vi "参数配置表.vi"() -> ()   [LabVIEW 2016, in "数据传输系统.lvlib"]
uses:
  <vilib>/Utility/miscctls.llb/LVPointTypeDef.ctl
  <vilib>/Utility/config.llb/NI_LVConfig.lvlib
  <vilib>/ptbypt/NI_PtbyPt.lvlib
panel:
  in  "应用环境":enum16{"STD", "GB212"}(ring)
  in  "屏蔽维护数据":bool
  in  "数据发送延时时间/s":i32
  in  "判断数据反馈":enum16{"非严格判断", "严格判断", "不判断"}(ring)
  in  "仪器参数发送":bool
  in  "地表水/污染源":bool
  in  "等时间间隔分钟":i32
  in  "数据发送通道":enum16{"TCP", "VISA"}(ring)
  in  "数据发送协议":enum16{"2005-212协议", "2017-212协议"}(ring)=enum."2017-212协议"
  in  "数据触发上传方式":enum16{"出数即刻发送", "等时间间隔定时发送", "整点发送"}(ring)
  in  "数据组合发送":bool
  in  "日志、参数发送":bool
  in  "2011发送":bool
  in  "返回":bool
  out "配置表格":string[][](table)
  in  "参数数值":T1={"CODMn"=TRUE, "CODCr"=TRUE, "DO"=TRUE, "铜"=TRUE, "PH"=TRUE, "氨氮"=TRUE, "比电导率"=TRUE, "水温"=TRUE, "COD"=TRUE, "浊度"=TRUE, "总氮"=TRUE, "总磷"=TRUE, "叶绿素a"=TRUE, "藻密度"=TRUE, "水位"=TRUE, "流速"=TRUE, "瞬时流量"=TRUE, "累积流量"=TRUE, "亚硝氮"=TRUE, "硫化物"=TRUE, "ORP"=TRUE, "铅"=TRUE, "镉"=TRUE, "锌"=TRUE, "镍"=TRUE, "锰"=TRUE, "汞"=TRUE, "气温"=TRUE, "气压"=TRUE, "风速"=TRUE, "风向"=TRUE}
  # "因子编码，单位配置，上传功能码，小时、质控数据上传触发方式"
  # "参数配置"
  # "只对2017版出数即刻发送有效"
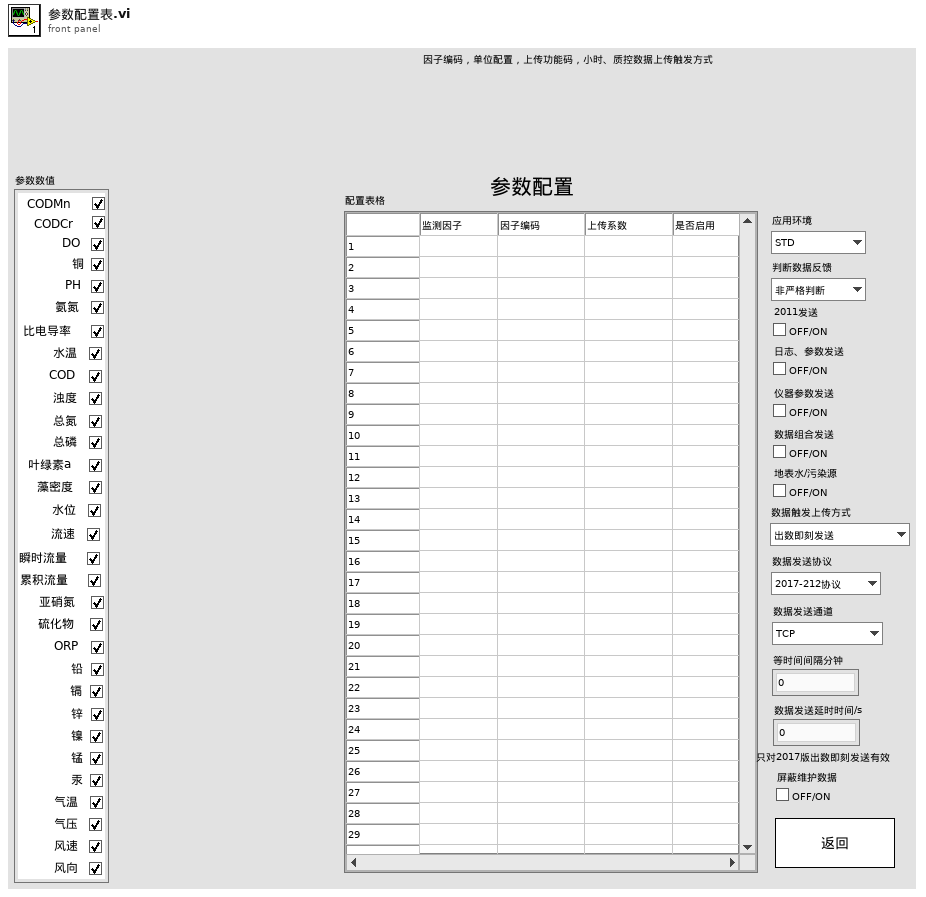
[diagram p1: front panel]
types:
  T1 = cluster{"CODMn":bool, "CODCr":bool, "DO":bool, "铜":bool, "PH":bool, "氨氮":bool, "比电导率":bool, "水温":bool, "COD":bool, "浊度":bool, "总氮":bool, "总磷":bool, "叶绿素a":bool, "藻密度":bool, "水位":bool, "流速":bool, "瞬时流量":bool, "累积流量":bool, "亚硝氮":bool, "硫化物":bool, "ORP":bool, "铅":bool, "镉":bool, "锌":bool, "镍":bool, "锰":bool, "汞":bool, "气温":bool, "气压":bool, "风速":bool, "风向":bool}
  T2 = typedef "LVPointTypeDef.ctl" = cluster{"Horizontal":i16, "Vertical":i16}
  T3 = typedef "NI_LVConfig.lvlib/Config Data RefNum.ctl" = refnum<k1>
  T4 = cluster{"[0]":string, "[1]":string, "[2]":string, "[3]":string, "[4]":string, "[5]":string, "[6]":string, "[7]":string, "[8]":string, "[9]":string, "[10]":string, "[11]":string, "[12]":string, "[13]":string, "[14]":string, "[15]":string, "[16]":string, "[17]":string, "[18]":string, "[19]":string, "[20]":string, "[21]":string, "[22]":string, "[23]":string, "[24]":string, "[25]":string, "[26]":string, "[27]":string, "[28]":string, "[29]":string, "[30]":string}
  T5 = enum8{"Enabled", "Disabled", "Disabled and Grayed Out"}
  T6 = typedef "LVRowAndColumnTypeDef.ctl" = cluster{"Row":i32, "Column":i32}
  T7 = cluster{"[0]":string, "[1]":string, "[2]":string, "[3]":string, "[4]":string, "[5]":string}
  T8 = cluster{"[0]":string, "[1]":string, "[2]":string, "[3]":string, "[4]":string, "[5]":string, "[6]":string, "[7]":string, "[8]":string, "[9]":string, "[10]":string, "[11]":string}
  T9 = cluster{"[0]":string, "[1]":string, "[2]":string, "[3]":string, "[4]":string, "[5]":string, "[6]":string, "[7]":string, "[8]":string, "[9]":string, "[10]":string, "[11]":string, "[12]":string}
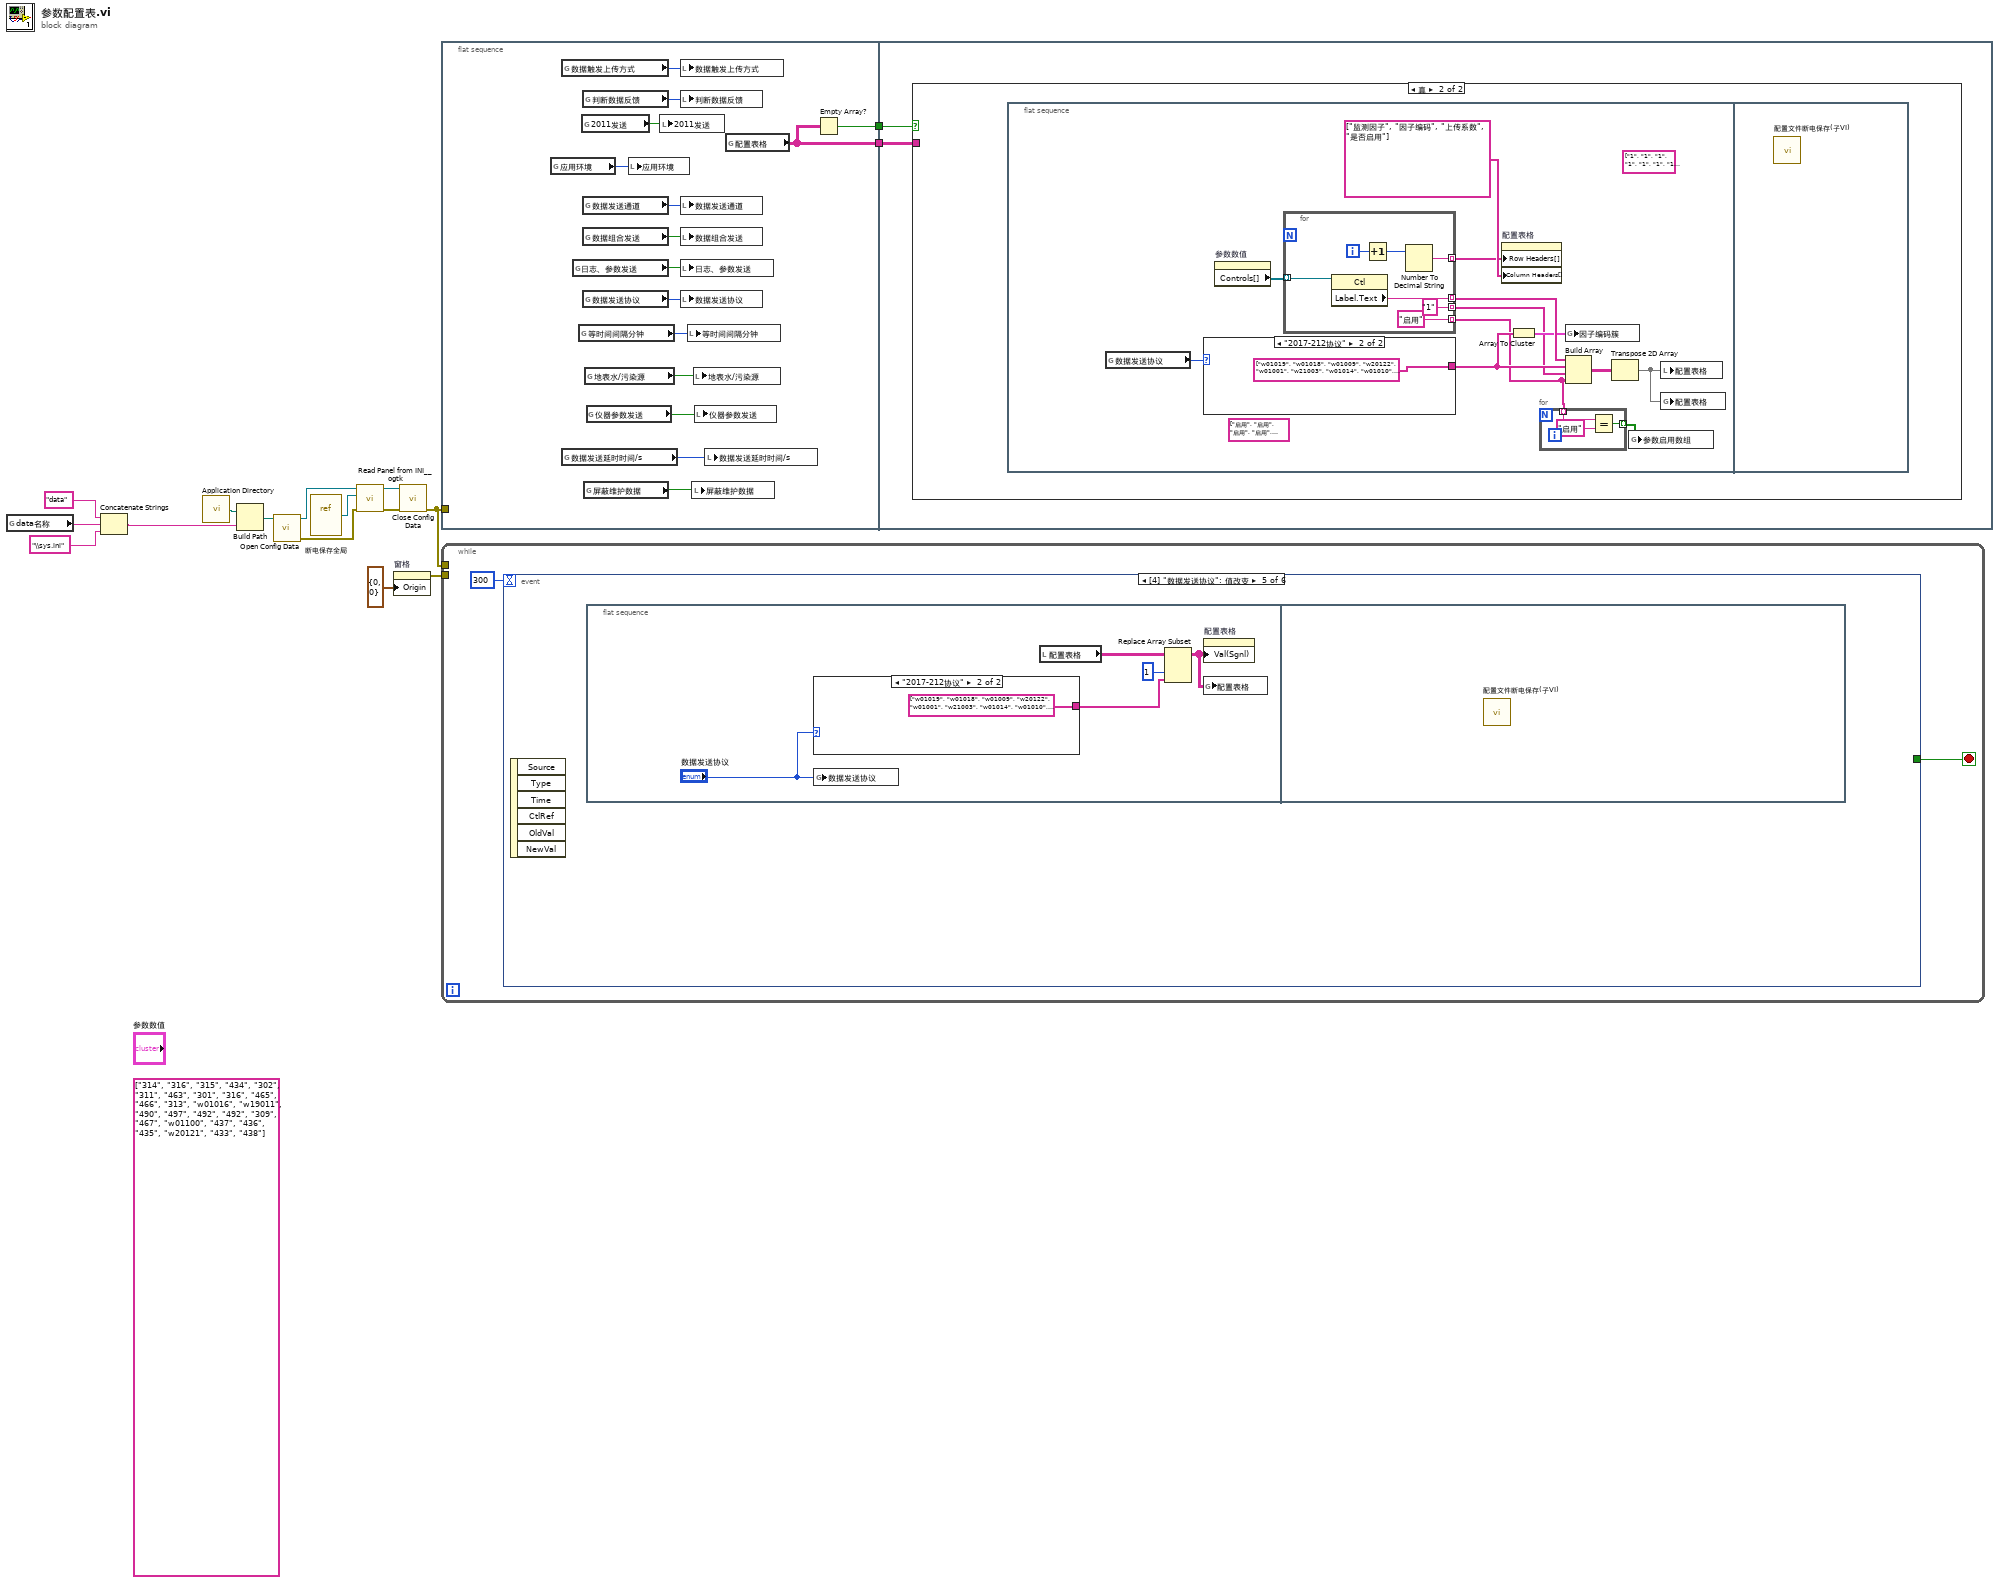
[diagram p0: block diagram]
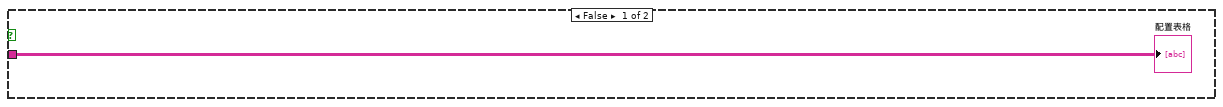
[diagram p2: hidden frame]
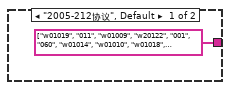
[diagram p3: hidden frame]
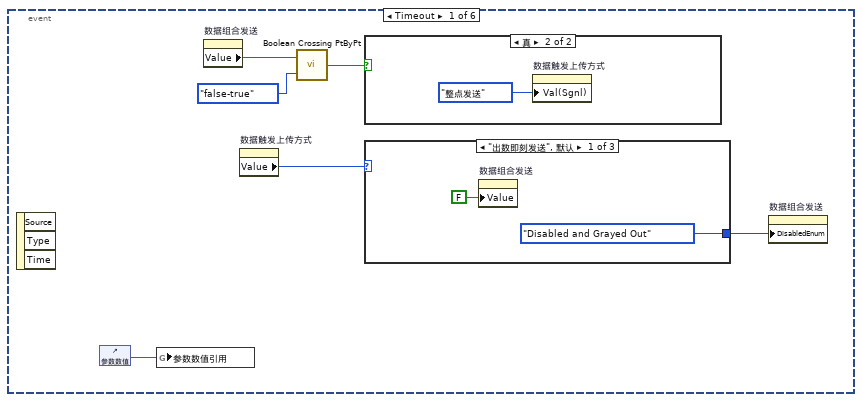
[diagram p4: hidden frame]
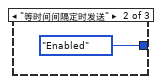
[diagram p6: hidden frame]
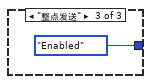
[diagram p7: hidden frame]
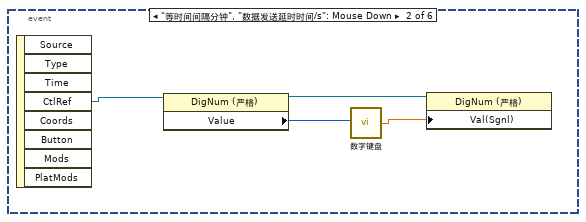
[diagram p8: hidden frame]
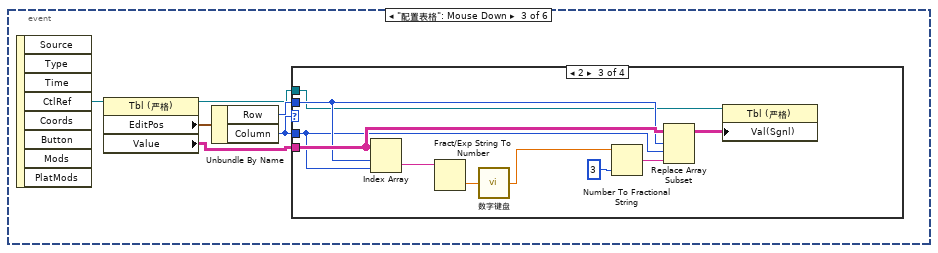
[diagram p9: hidden frame]
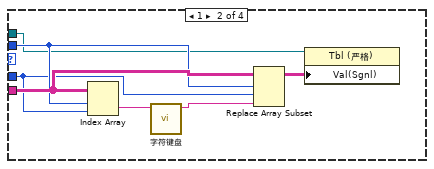
[diagram p11: hidden frame]
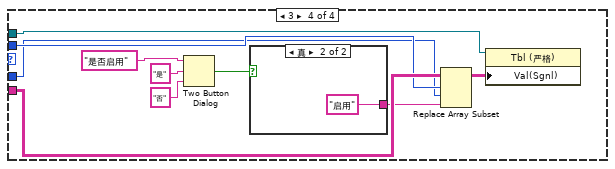
[diagram p12: hidden frame]
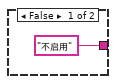
[diagram p13: hidden frame]
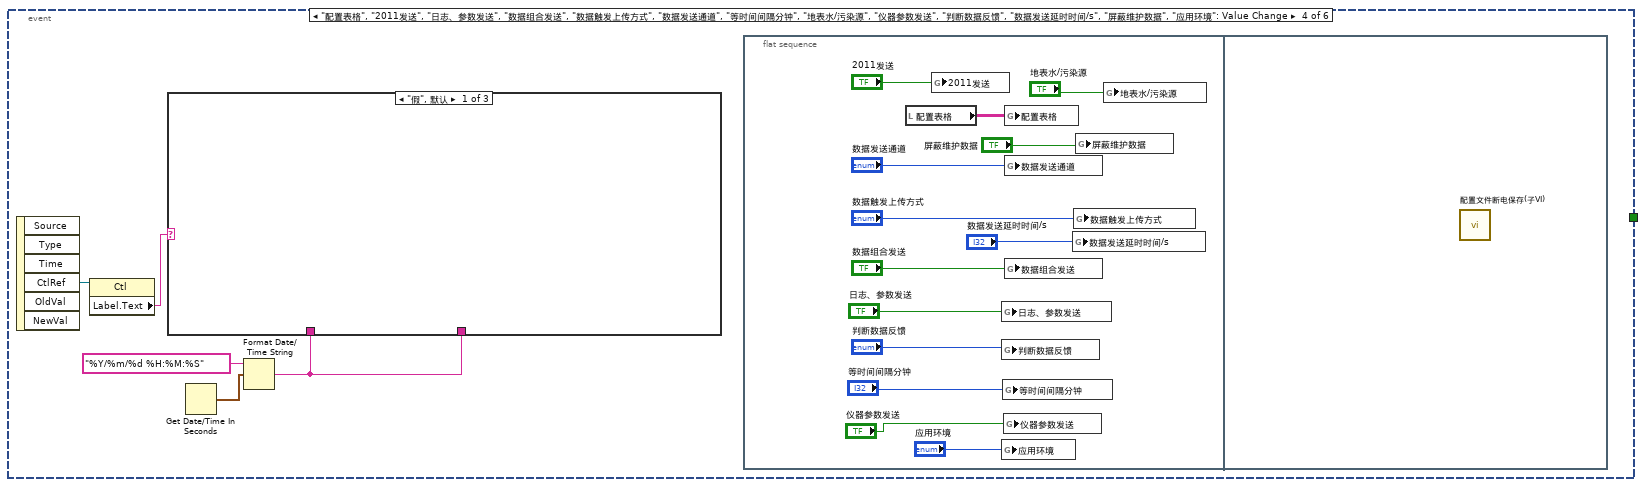
[diagram p14: hidden frame]
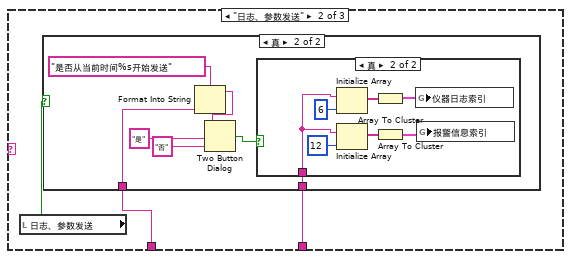
[diagram p15: hidden frame]
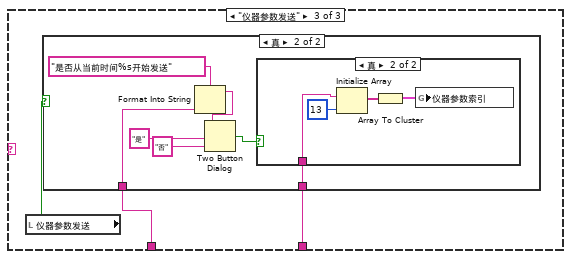
[diagram p18: hidden frame]
diagram:
  (unwired) string[] ["314", "316", "315", "434", "302", "311", "463", "301", "316", "465", "466", "313", "w01016", "w19011", "490", "497", "492", "492", "309", "467", "w01100", "437", "436", "435", "w20121", "433", "438"]
  n1 = global read "断电保存全局.vi" "data名称"() -> (w3:string)
  n2 = Concatenate Strings("data" ("名称或相对路径"), w3, "\\sys.ini" ("名称或相对路径")) -> (w1:string)
  n3 = call <vilib>:"Application Directory.vi"() -> ("Application Directory"=w12:path)
  n4 = Build Path(base path=w12, name or relative path=w1) -> (appended path=w11:path)
  n5 = call <vilib>:"Open Config Data.vi"("configuration file path"=w11) -> ("error out"=w16:errorcluster, "refnum"=w15:T3)  [unwired: 8 in, 1 out]
  n6 = vi-ref "断电保存全局.vi"() -> (w14:refnum<vi>)
  n7 = call <userlib>:"Read Panel from INI__ogtk.vi"("error in (no error)"=w16, "VI ref"=w14, "refnum"=w15) -> ("error out"=w10:errorcluster, "refnum out"=w13:T3)  [unwired: 7 in]
  n8 = property on="窗格" class="Pane"("Origin"=T2 {"Horizontal"=0, "Vertical"=0} ("原点")) -> (error out=w8:errorcluster)  [unwired: 2 in, 1 out]
  n9 = call <vilib>:"Close Config Data.vi"("error in (no error)"=w10, "refnum"=w13) -> ("error out"=w9:errorcluster)  [unwired: 8 in, 1 out]
  n10 = flat-sequence {
    tunnel: w9 -> [_]
    tunnel: [w24] -> w6
    tunnel: [w23] -> w5
    tunnel: w6 -> [w33]
    tunnel: w5 -> [w32]
    frame #0 {
      n11 = global read "断电保存全局.vi" "应用环境"() -> (w17:enum16{"STD", "GB212"})
      n12 = global read "断电保存全局.vi" "数据触发上传方式"() -> (w27:enum16{"出数即刻发送", "等时间间隔定时发送", "整点发送"})
      n13 = global read "断电保存全局.vi" "数据发送延时时间/s"() -> (w19:i32)
      n14 = global read "断电保存全局.vi" "日志、参数发送"() -> (w29:bool)
      n15 = global read "断电保存全局.vi" "等时间间隔分钟"() -> (w22:i32)
      n16 = global read "断电保存全局.vi" "2011发送"() -> (w31:bool)
      n17 = global read "断电保存全局.vi" "判断数据反馈"() -> (w30:enum16{"非严格判断", "严格判断", "不判断"})
      n18 = global read "断电保存全局.vi" "数据发送通道"() -> (w26:enum16{"TCP", "VISA"})
      n19 = global read "断电保存全局.vi" "数据组合发送"() -> (w28:bool)
      n20 = global read "断电保存全局.vi" "数据发送协议"() -> (w25:enum16{"2005-212协议", "2017-212协议"})
      n21 = global read "断电保存全局.vi" "屏蔽维护数据"() -> (w18:bool)
      n22 = global read "断电保存全局.vi" "地表水/污染源"() -> (w21:bool)
      n23 = global read "断电保存全局.vi" "仪器参数发送"() -> (w20:bool)
      n24 = local write "应用环境"(w17) -> ()
      n25 = local write "2011发送"(w31) -> ()
      n26 = local write "数据触发上传方式"(w27) -> ()
      n27 = local write "判断数据反馈"(w30) -> ()
      n28 = local write "数据发送通道"(w26) -> ()
      n29 = local write "数据组合发送"(w28) -> ()
      n30 = local write "日志、参数发送"(w29) -> ()
      n31 = local write "数据发送协议"(w25) -> ()
      n32 = local write "等时间间隔分钟"(w22) -> ()
      n33 = local write "屏蔽维护数据"(w18) -> ()
      n34 = local write "地表水/污染源"(w21) -> ()
      n35 = local write "仪器参数发送"(w20) -> ()
      n36 = local write "数据发送延时时间/s"(w19) -> ()
      n37 = global read "断电保存全局.vi" "配置表格"() -> (w23:string[][])
      n38 = Empty Array?(array=w23) -> (empty?=w24:bool)
    }
    frame #1 {
      n39 = case shown="真" w33 {
        tunnel: w32 -> [w34 _]
        frame False {
          "配置表格" <- w34
        }
        frame True {
          n40 = flat-sequence {
            frame #0 {
              (unwired) string[] ["启用", "启用", "启用", "启用", "启用", "启用", "启用", "启用", "启用", "启用", "启用", "启用", "启用", "启用", "启用", "启用", "启用", "启用", "启用", "启用", "启用", "启用", "启用", "启用", "启用", "启用", "启用"]
              (unwired) string[] ["1", "1", "1", "1", "1", "1", "1", "1", "1", "1", "1", "1", "1", "1", "1", "1", "1", "1", "1", "1", "1", "1", "1", "1", "1", "1", "1"]
              n41 = global read "断电保存全局.vi" "数据发送协议"() -> (w40:enum16{"2005-212协议", "2017-212协议"})
              n42 = case shown="\"2017-212协议\"" w40 {
                tunnel: [string[] ["w01019", "011", "w01009", "w20122", "001", "060", "w01014", "w01010", "w01018", "w01003", "065", "101", "w01016", "w19011", "e01201", "e01202", "B01", "e01204", "w21006", "w21019", "w01100", "w20120", "w20115", "w20123", "w20121", "w20124", "w20111"] string[] ["w01019", "w01018", "w01009", "w20122", "w01001", "w21003", "w01014", "w01010", "w01018", "w01003", "w21001", "w21011", "w01016", "w19011", "e01201", "e01202", "e01203", "e01204", "w21006", "w21019", "w01100", "w20120", "w20115", "w20123", "w20121", "w20124", "w20111", "a01001", "a01006", "a01007", "a01008"]] -> w38
                frame "2005-212协议", Default {
                }
                frame "2017-212协议" {
                }
              }
              n43 = property on="参数数值" class="Clust (严格)"() -> ("Controls[]"=w42:refnum<vi>[])  [unwired: 2 in, 2 out]
              n44 = for {
                tunnel: w42 -> [w58] mode=indexing
                tunnel: [w57] -> w44 mode=indexing
                tunnel: [w55] -> w43 mode=indexing
                tunnel: ["1"] -> w37 mode=indexing
                tunnel: ["启用"] -> w35 mode=indexing
                i -> [w56]
                n45 = property class="Ctl"(reference=w58) -> ("Label.Text"=w57:string)  [unwired: 1 in, 2 out]
                n46 = Increment(x=w56) -> (x+1=w54:i32)
                n47 = Number To Decimal String(number=w54) -> (decimal integer string=w55:string)  [unwired: 1 in]
              }
              n48 = property on="配置表格" class="Tbl (严格)"("Row Headers[]"=w43, "Column Headers[]"=string[] ["监测因子", "因子编码", "上传系数", "是否启用"]) -> ()  [unwired: 2 in, 2 out]
              n49 = Array To Cluster(array=w38) -> (cluster=w39:T4)
              n50 = for {
                tunnel: w35 -> [w49] mode=indexing
                tunnel: [w47] -> w36 mode=indexing
                n51 = Equal?(x=w49, y="启用") -> (x = y?=w47:bool)
              }
              n52 = global write "断电保存全局.vi" "因子编码簇"(w39) -> ()
              n53 = Build Array(w44, w38, w37, w35) -> (w46:string[][])
              n54 = Transpose 2D Array(2D array=w46) -> (transposed array=w41:string[][])
              n55 = global write "断电保存全局.vi" "参数启用数组"(w36) -> ()
              n56 = local write "配置表格"(w41) -> ()
              n57 = global write "断电保存全局.vi" "配置表格"(w41) -> ()
            }
            frame #1 {
              n58 = call "配置文件断电保存(子VI).vi"() -> ()  [unwired: 12 in]
            }
          }
        }
      }
    }
  }
  n59 = while {
    tunnel: w9 -> [_]
    tunnel: w8 -> [_]
    stop <- w59 stop-if-true
    n60 = event shown="[4] \"数据发送协议\": 值改变" {
      selector: _ -> [_ _ _ _ _ _]
      dyn-events: _ -> [_ _ _ _ _ _]
      timeout: 300 -> [_ _ _ _ _ _]
      tunnel: [_ _ _ _ _ TRUE] -> w59
      event Timeout {
        n61 = event-data() -> ()  [unwired: 1 in, 3 out]
        n62 = control-ref of="参数数值"() -> (w61:refnum<vi>)
        n63 = global write "断电保存全局.vi" "参数数值引用"(w61) -> ()
        n64 = property on="数据组合发送" class="Bool (严格)"() -> ("Value"=w64:bool)  [unwired: 2 in, 2 out]
        n65 = property on="数据触发上传方式" class="Enum (严格)"() -> ("Value"=w66:enum16{"出数即刻发送", "等时间间隔定时发送", "整点发送"})  [unwired: 2 in, 2 out]
        n66 = call <vilib>:"Boolean Crossing PtByPt.vi"("direction"=enum16{"either", "false-true", "true-false"}."false-true", "input"=w64) -> ("crossing"=w62:bool)  [unwired: 1 in]
        n67 = case shown="真" w62 {
          frame False {
          }
          frame True {
            n68 = property on="数据触发上传方式" class="Enum (严格)"("Val(Sgnl)"=enum16{"出数即刻发送", "等时间间隔定时发送", "整点发送"}."整点发送" ("值(信号)")) -> ()  [unwired: 2 in, 2 out]
          }
        }
        n69 = case shown="\"出数即刻发送\", 默认" w66 {
          tunnel: [T5."Disabled and Grayed Out" ("禁用") T5."Enabled" ("禁用") T5."Enabled" ("禁用")] -> w65
          frame "出数即刻发送", Default {
            n70 = property on="数据组合发送" class="Bool (严格)"("Value"=FALSE ("值(信号)")) -> ()  [unwired: 2 in, 2 out]
          }
          frame "等时间间隔定时发送" {
          }
          frame "整点发送" {
          }
        }
        n71 = property on="数据组合发送" class="Bool (严格)"("DisabledEnum"=w65) -> ()  [unwired: 2 in, 2 out]
      }
      event "等时间间隔分钟", "数据发送延时时间/s": Mouse Down {
        n72 = event-data() -> ("CtlRef"=w75:refnum<vi>)  [unwired: 1 in, 7 out]
        n73 = property class="DigNum (严格)"(reference=w75) -> (reference out=w73:refnum<vi>, "Value"=w74:i32)  [unwired: 1 in, 1 out]
        n74 = call "数字键盘.vi"("OldNumber"=w74) -> ("NewNumber"=w72:sgl)
        n75 = property class="DigNum (严格)"(reference=w73, "Val(Sgnl)"=w72) -> ()  [unwired: 1 in, 2 out]
      }
      event "配置表格": Mouse Down {
        n76 = event-data() -> ("CtlRef"=w81:refnum<vi>)  [unwired: 1 in, 7 out]
        n77 = property class="Tbl (严格)"(reference=w81) -> (reference out=w77:refnum<vi>, "EditPos"=w80:T6, "Value"=w79:string[][])  [unwired: 1 in, 1 out]
        n78 = Unbundle By Name(w80) -> ("Row"=w78:i32, "Column"=w76:i32)
        n79 = case shown="2" w76 {
          tunnel: w79 -> [_ w87 w98 w102]
          tunnel: w78 -> [_ w86 w97 w101]
          tunnel: w76 -> [_ w85 w96 w100]
          tunnel: w77 -> [_ w83 w95 w103]
          frame 0, Default {
          }
          frame 1 {
            n80 = Index Array(array=w87, index (row)=w86, index (col)=w85) -> (element=w88:string)
            n81 = call "字符键盘.vi"("原值"=w88) -> ("x+y"=w84:string)  [unwired: 10 in]
            n82 = Replace Array Subset(array=w87, new element=w84, index (row)=w86, index (col)=w85) -> (w82:string[][])
            n83 = property class="Tbl (严格)"(reference=w83, "Val(Sgnl)"=w82) -> ()  [unwired: 1 in, 2 out]
          }
          frame 2 {
            n84 = Index Array(array=w98, index (row)=w97, index (col)=w96) -> (element=w93:string)
            n85 = Fract/Exp String To Number(string=w93) -> (number=w92:dbl)  [unwired: 3 in, 1 out]
            n86 = call "数字键盘.vi"("OldNumber"=w92) -> ("NewNumber"=w91:sgl)
            n87 = Number To Fractional String(number=w91, precision (6)=i16 3 ("精度(6)")) -> (F-format string=w90:string)  [unwired: 2 in]
            n88 = Replace Array Subset(array=w98, new element=w90, index (row)=w97, index (col)=w96) -> (w94:string[][])
            n89 = property class="Tbl (严格)"(reference=w95, "Val(Sgnl)"=w94) -> ()  [unwired: 1 in, 2 out]
          }
          frame 3 {
            n90 = Two Button Dialog(message="是否启用" ("消息"), 1:"否" ("F按钮名称（“取消”）"), 2:"是" ("T按钮名称（“确定”）")) -> (T button?=w105:bool)
            n91 = case shown="真" w105 {
              tunnel: ["不启用" "启用"] -> w99
              frame False {
              }
              frame True {
              }
            }
            n92 = Replace Array Subset(array=w102, new element=w99, index (row)=w101, index (col)=w100) -> (w104:string[][])
            n93 = property class="Tbl (严格)"(reference=w103, "Val(Sgnl)"=w104) -> ()  [unwired: 1 in, 2 out]
          }
        }
      }
      event "配置表格", "2011发送", "日志、参数发送", "数据组合发送", "数据触发上传方式", "数据发送通道", "等时间间隔分钟", "地表水/污染源", "仪器参数发送", "判断数据反馈", "数据发送延时时间/s", "屏蔽维护数据", "应用环境": Value Change {
        n94 = event-data() -> ("CtlRef"=w115:refnum<vi>)  [unwired: 1 in, 5 out]
        n95 = property class="Ctl"(reference=w115) -> ("Label.Text"=w114:string)  [unwired: 1 in, 2 out]
        n96 = Get Date/Time In Seconds() -> (seconds since 1Jan1904=w113:timestamp)
        n97 = Format Date/Time String(time format string (%c)="%Y/%m/%d %H:%M:%S" ("时间格式字符串(%c)"), seconds (now)=w113) -> (date/time string=w111:string)  [unwired: 1 in]
        n98 = case shown="\"假\", 默认" w114 {
          tunnel: w111 -> [_ w117 w134]
          tunnel: w111 -> [_ w116 w133]
          frame "假", Default {
          }
          frame "日志、参数发送" {
            n99 = local read "日志、参数发送"() -> (w118:bool)
            n100 = case shown="真" w118 {
              tunnel: w117 -> [_ w122]
              tunnel: w116 -> [_ w120]
              frame False {
              }
              frame True {
                n101 = Format Into String(format string="是否从当前时间%s开始发送" ("消息"), w120) -> (resulting string=w119:string)  [unwired: 2 in, 1 out]
                n102 = Two Button Dialog(message=w119, 1:"否" ("F按钮名称（“取消”）"), 2:"是" ("T按钮名称（“确定”）")) -> (T button?=w123:bool)
                n103 = case shown="真" w123 {
                  tunnel: w122 -> [_ w126]
                  frame False {
                  }
                  frame True {
                    n104 = Initialize Array(w126, 6 ("维数大小")) -> (w132:string[])
                    n105 = Initialize Array(w126, 12 ("维数大小")) -> (w128:string[])
                    n106 = Array To Cluster(array=w132) -> (cluster=w130:T7)
                    n107 = Array To Cluster(array=w128) -> (cluster=w127:T8)
                    n108 = global write "全局 时间2.vi" "仪器日志索引"(w130) -> ()
                    n109 = global write "全局 时间2.vi" "报警信息索引"(w127) -> ()
                  }
                }
              }
            }
          }
          frame "仪器参数发送" {
            n110 = local read "仪器参数发送"() -> (w135:bool)
            n111 = case shown="真" w135 {
              tunnel: w134 -> [_ w139]
              tunnel: w133 -> [_ w137]
              frame False {
              }
              frame True {
                n112 = Format Into String(format string="是否从当前时间%s开始发送" ("消息"), w137) -> (resulting string=w136:string)  [unwired: 2 in, 1 out]
                n113 = Two Button Dialog(message=w136, 1:"否" ("F按钮名称（“取消”）"), 2:"是" ("T按钮名称（“确定”）")) -> (T button?=w140:bool)
                n114 = case shown="真" w140 {
                  tunnel: w139 -> [_ w143]
                  frame False {
                  }
                  frame True {
                    n115 = Initialize Array(w143, 13 ("维数大小")) -> (w146:string[])
                    n116 = Array To Cluster(array=w146) -> (cluster=w144:T9)
                    n117 = global write "全局 时间2.vi" "仪器参数索引"(w144) -> ()
                  }
                }
              }
            }
          }
        }
        n118 = flat-sequence {
          frame #0 {
            n119 = local read "配置表格"() -> (w159:string[][])
            n120 = global write "断电保存全局.vi" "2011发送"("2011发送") -> ()
            n121 = global write "断电保存全局.vi" "日志、参数发送"("日志、参数发送") -> ()
            n122 = global write "断电保存全局.vi" "判断数据反馈"("判断数据反馈") -> ()
            n123 = global write "断电保存全局.vi" "应用环境"("应用环境") -> ()
            n124 = global write "断电保存全局.vi" "等时间间隔分钟"("等时间间隔分钟") -> ()
            n125 = global write "断电保存全局.vi" "仪器参数发送"("仪器参数发送") -> ()
            n126 = global write "断电保存全局.vi" "配置表格"(w159) -> ()
            n127 = global write "断电保存全局.vi" "数据发送通道"("数据发送通道") -> ()
            n128 = global write "断电保存全局.vi" "数据组合发送"("数据组合发送") -> ()
            n129 = global write "断电保存全局.vi" "数据发送延时时间/s"("数据发送延时时间/s") -> ()
            n130 = global write "断电保存全局.vi" "数据触发上传方式"("数据触发上传方式") -> ()
            n131 = global write "断电保存全局.vi" "屏蔽维护数据"("屏蔽维护数据") -> ()
            n132 = global write "断电保存全局.vi" "地表水/污染源"("地表水/污染源") -> ()
          }
          frame #1 {
            n133 = call "配置文件断电保存(子VI).vi"() -> ()  [unwired: 12 in]
          }
        }
      }
      event "数据发送协议": Value Change {
        n134 = event-data() -> ()  [unwired: 1 in, 6 out]
        n135 = flat-sequence {
          frame #0 {
            n136 = case shown="\"2017-212协议\"" "数据发送协议" {
              tunnel: [string[] ["w01019", "011", "w01009", "w20122", "001", "060", "w01014", "w01010", "w01018", "w01003", "065", "101", "w01016", "w19011", "e01201", "e01202", "B01", "e01204", "w21006", "w21019", "w01100", "w20120", "w20115", "w20123", "w20121", "w20124", "w20111"] string[] ["w01019", "w01018", "w01009", "w20122", "w01001", "w21003", "w01014", "w01010", "w01018", "w01003", "w21001", "w21011", "w01016", "w19011", "e01201", "e01202", "e01203", "e01204", "w21006", "w21019", "w01100", "w20120", "w20115", "w20123", "w20121", "w20124", "w20111"]] -> w162
              frame "2005-212协议", Default {
              }
              frame "2017-212协议" {
              }
            }
            n137 = global write "断电保存全局.vi" "数据发送协议"("数据发送协议") -> ()
            n138 = local read "配置表格"() -> (w163:string[][])
            n139 = Replace Array Subset(array=w163, new element=w162, index (col)=1 ("禁用的索引 (列)")) -> (w160:string[][])  [unwired: 1 in]
            n140 = property on="配置表格" class="Tbl (严格)"("Val(Sgnl)"=w160) -> ()  [unwired: 2 in, 2 out]
            n141 = global write "断电保存全局.vi" "配置表格"(w160) -> ()
          }
          frame #1 {
            n142 = call "配置文件断电保存(子VI).vi"() -> ()  [unwired: 12 in]
          }
        }
      }
      event "返回": Value Change; Panel Close {
        n143 = event-data() -> ()  [unwired: 1 in, 3 out]
      }
    }
  }
